vi "Send Message.vi"(8 "error in":errorcluster, 10 "IMessage":refnum<class "IMessage.lvclass">, 11 "PCAN Basic Read-Write CAN Frame Strategy in":refnum<class "PCAN Basic Read-Write CAN Frame Strategy.lvclass">) -> (0 "error out":errorcluster, 3 "PCAN Basic Read-Write CAN Frame Strategy out":refnum<class "PCAN Basic Read-Write CAN Frame Strategy.lvclass">)   [LabVIEW 2025, in "PCAN Basic Read-Write CAN Frame Strategy.lvclass"]
uses:
  PCAN Basic Read-Write CAN Frame Strategy.lvclass
  Source/Interfaces/IMessage/IMessage.lvclass
  <instrlib>/Peter/PCAN Basic/PCAN Message.ctl
  <instrlib>/Peter/PCAN Basic/PCAN Message types.ctl
  <instrlib>/Peter/PCAN Basic/PCANBasic.lvlib
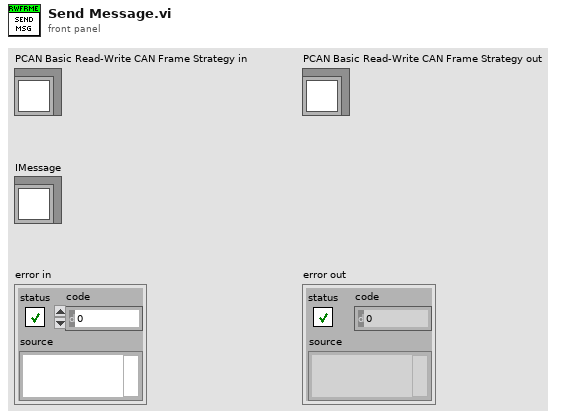
[diagram p1: front panel]
types:
  T1 = typedef "PCANBasic.lvlib/PCAN Message.ctl" = cluster{"ID":u32, "MSGTYPE":T2, "LEN":u8, "DATA":cluster{"0":u8, "1":u8, "2":u8, "3":u8, "4":u8, "5":u8, "6":u8, "7":u8}}
  T2 = typedef "PCANBasic.lvlib/PCAN Message types.ctl" = u8
  T3 = cluster{"Data[0]":u8, "Data[1]":u8, "Data[2]":u8, "Data[3]":u8, "Data[4]":u8, "Data[5]":u8, "Data[6]":u8, "Data[7]":u8}
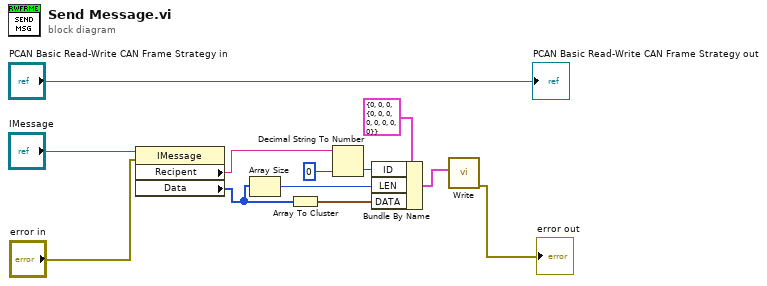
[diagram p0: block diagram]
diagram:
  n1 = property class="IMessage"(reference="IMessage", error in="error in") -> ("Recipent"=w4:string, "Data"=w2:u8[])  [unwired: 2 out]
  n2 = Array Size(array=w2) -> (size(s)=w1:i32)
  n3 = Array To Cluster(array=w2) -> (cluster=w3:T3)
  n4 = Decimal String To Number(string=w4, default (0L)=u32 0) -> (number=w5:u32)  [unwired: 1 in, 1 out]
  n5 = Bundle By Name(cluster=T1 {"ID"=0, "MSGTYPE"=0, "LEN"=0, "DATA"={"0"=0, "1"=0, "2"=0, "3"=0, "4"=0, "5"=0, "6"=0, "7"=0}} ("PCAN Message"), "ID"=w5, "LEN"=w1, "DATA"=w3) -> (w7:T1)
  n6 = call <instrlib>:"Write.vi"("PCAN Message"=w7) -> ("error out"=→"error out":errorcluster)  [unwired: 8 in, 2 out]
  "PCAN Basic Read-Write CAN Frame Strategy out" <- "PCAN Basic Read-Write CAN Frame Strategy in"
